vi "findIndex.vi"(10 "Disp.":u8, 11 "Acc.":u8) -> (3 "Index":u8)   [LabVIEW 2019]
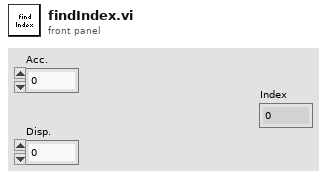
[diagram p1: front panel]
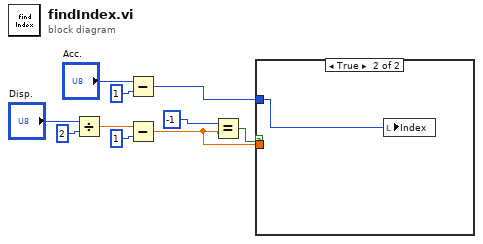
[diagram p0: block diagram]
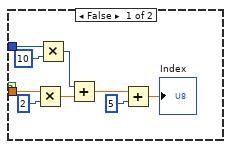
[diagram p2: hidden frame]
diagram:
  n1 = Divide(x="Disp.", y=2) -> (x/y=w10:dbl)
  n2 = Subtract(x="Acc.", y=1) -> (x-y=w4:i32)
  n3 = Subtract(x=w10, y=1) -> (x-y=w1:dbl)
  n4 = Equal?(x=-1, y=w1) -> (x = y?=w3:bool)
  n5 = case shown="True" w3 {
    tunnel: w1 -> [w17 _]
    tunnel: w4 -> [w11 w20]
    frame False {
      n6 = Multiply(x=w17, y=2) -> (x*y=w19:dbl)
      n7 = Multiply(x=w11, y=10) -> (x*y=w18:i32)
      n8 = Add(x=w18, y=w19) -> (x+y=w14:dbl)
      n9 = Add(x=w14, y=5) -> (x+y=→"Index":dbl)
    }
    frame True {
      n10 = local write "Index"(w20) -> ()
    }
  }
